vi "Pre Launch Init.vi"(11 "Nested in":refnum<class "Object Dictionary UI.lvclass">) -> (0 "error out":errorcluster, 3 "Nested out":refnum<class "Object Dictionary UI.lvclass">)   [LabVIEW 2020, in "Object Dictionary UI.lvlib" / "Object Dictionary UI.lvclass"]
doc: "(<B>Filename</B>: Actor Framework.lvlib:Actor.lvclass:Pre Launch Init.vi)\n\nDefines behavior that occurs after the Launch Nested Actor method is invoked but before the actor's Actor Core method begins running.\n\nBy default, this method does nothing. A descendant class may override it to define behavior."
uses:
  Object Dictionary UI.lvclass
  Object Dictionary UI.lvclass/Object Dictionary UI.ctl
  <vilib>/MGI/Panel Manager/Panel Actor/Panel Actor/Panel Actor.lvclass
  source/Typedefs/Access SRDO.ctl
  source/CANopen.lvlib
  source/Typedefs/Access PDO.ctl
  source/Typedefs/Access SDO.ctl
  source/Typedefs/Object Type.ctl
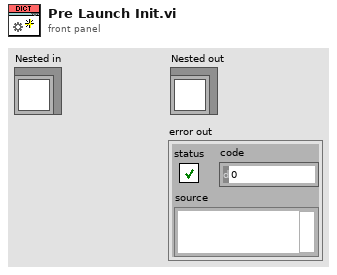
[diagram p1: front panel]
types:
  T1 = typedef "CANopen.lvlib/Object Type.ctl" = u8
  T2 = typedef "CANopen.lvlib/Access SDO.ctl" = enum16{"read only", "write only", "read/write", "read/write on process input", "read/write on process output", "constant value", "no", "UNKNOWN"}
  T3 = typedef "CANopen.lvlib/Access PDO.ctl" = enum16{"no", "TPDO", "RPDO", "TPDO & RPDO"}
  T4 = typedef "CANopen.lvlib/Access SRDO.ctl" = enum16{"no", "tx", "rx", "trx"}
  T5 = cluster{"Index":string, "Sub-Index":string, "ParameterName":string, "Denotation":string, "Description":string, "ObjectType":T1, "HighLimit":string, "DataType":u16, "LowLimit":string, "Access SDO":T2, "Access PDO":T3, "Access SRDO":T4, "DefaultValue":string}
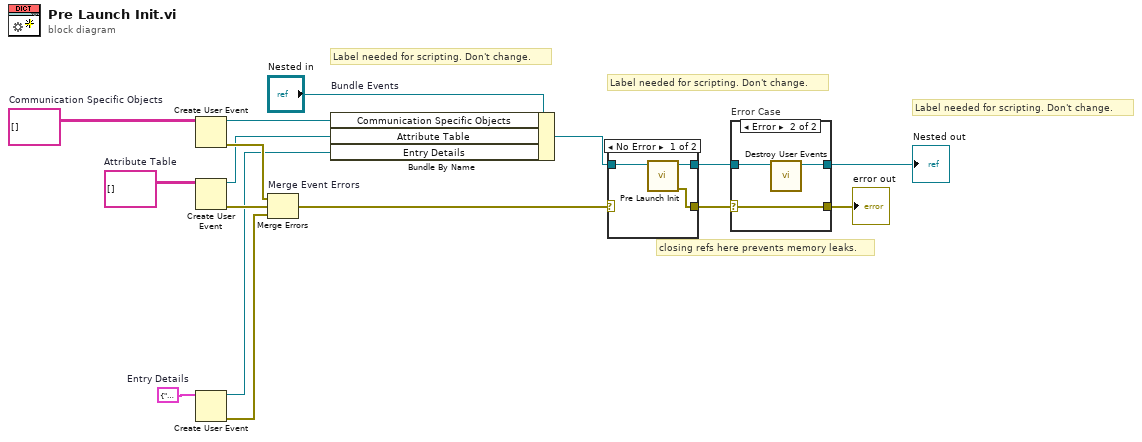
[diagram p0: block diagram]
diagram:
  w3 = T5 {"Index"="", "Sub-Index"="", "ParameterName"="", "Denotation"="", "Description"="", "ObjectType"=0, "HighLimit"="", "DataType"=0, "LowLimit"="", "Access SDO"=enum."read only", "Access PDO"=enum."no", "Access SRDO"=enum."no", "DefaultValue"=""}  # Entry Details
  w6 = string[][] []  # Attribute Table
  w8 = string[][] []  # Communication Specific Objects
  # "Label needed for scripting. Don't change."
  # "Label needed for scripting. Don't change."
  # "Label needed for scripting. Don't change."
  # "closing refs here prevents memory leaks."
  n1 = Create User Event(user event datatype=w8) -> (user event=w7:refnum<user-event>, error out=w15:errorcluster)  [unwired: 1 in]
  n2 = Create User Event(user event datatype=w6) -> (user event=w5:refnum<user-event>, error out=w4:errorcluster)  [unwired: 1 in]
  n3 = Create User Event(user event datatype=w3) -> (user event=w2:refnum<user-event>, error out=w1:errorcluster)  [unwired: 1 in]
  n4 = Merge Errors "Merge Event Errors"(w15, w4, w1) -> (w10:errorcluster)
  n5 = Bundle By Name "Bundle Events"(cluster="Nested in", "Communication Specific Objects"=w7, "Attribute Table"=w5, "Entry Details"=w2) -> (w11:refnum<class "Object Dictionary UI.lvclass">)
  n6 = case shown="No Error" w10 {
    selector: w10 -> [_ w21]
    tunnel: [w19 w20] -> w12
    tunnel: w11 -> [w18 w20]
    tunnel: [w17 w21] -> w9
    frame No Error {
      n7 = call-parent "Pre Launch Init.vi"("Panel Actor in"=w18) -> ("error out"=w17:errorcluster, "Panel Actor out"=w19:refnum<class "Object Dictionary UI.lvclass">)  [unwired: 9 in]
    }
    frame Error {
    }
  }
  n8 = case "Error Case" shown="Error" w9 {
    selector: w9 -> [w22 w26]
    tunnel: w12 -> [w23 w25]
    tunnel: [w23 w24] -> w14
    tunnel: [w22 w26] -> w13
    frame No Error {
    }
    frame Error {
      n9 = call "Destroy User Events.vi"("UI Template in"=w25) -> ("UI Template out"=w24:refnum<class "Object Dictionary UI.lvclass">)  [unwired: 10 in]
    }
  }
  "error out" <- w13
  "Nested out" <- w14
